vi "GetControlRef[Poly].vi"   [LabVIEW 2016]
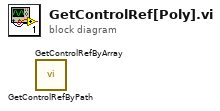
[diagram p0: block diagram]
diagram:
  n1 = call "GetControlRefByPath.vi"() -> ()  [unwired: 13 in, 3 out]
  n2 = call "GetControlRefByArray.vi"() -> ()  [unwired: 13 in, 3 out]
